vi "TRAMAGGA.vi"(0 "TRAMA":string) -> (1 "Cluster 2":T2, 2 "Cluster":T3, 3 "Cluster 3":T1, 4 "String":string)   [LabVIEW 2020]
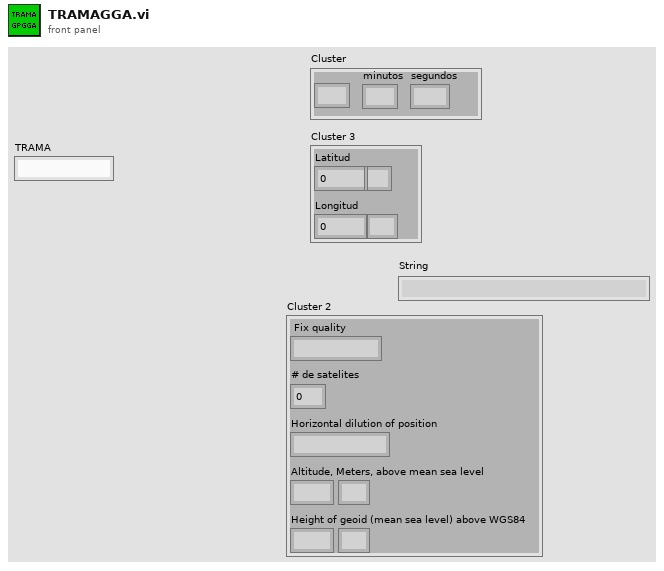
[diagram p1: front panel]
types:
  T1 = cluster{"Latitud":dbl, string, "Longitud":dbl, string}
  T2 = cluster{" Fix quality":string, "# de satelites":dbl, "Horizontal dilution of position":string, "Altitude, Meters, above mean sea level":string, string, "Height of geoid (mean sea level) above WGS84":string, string}
  T3 = cluster{"horas":string, "minutos":string, "segundos ":string}
  T4 = cluster{string, dbl, string, string, string, string, string}
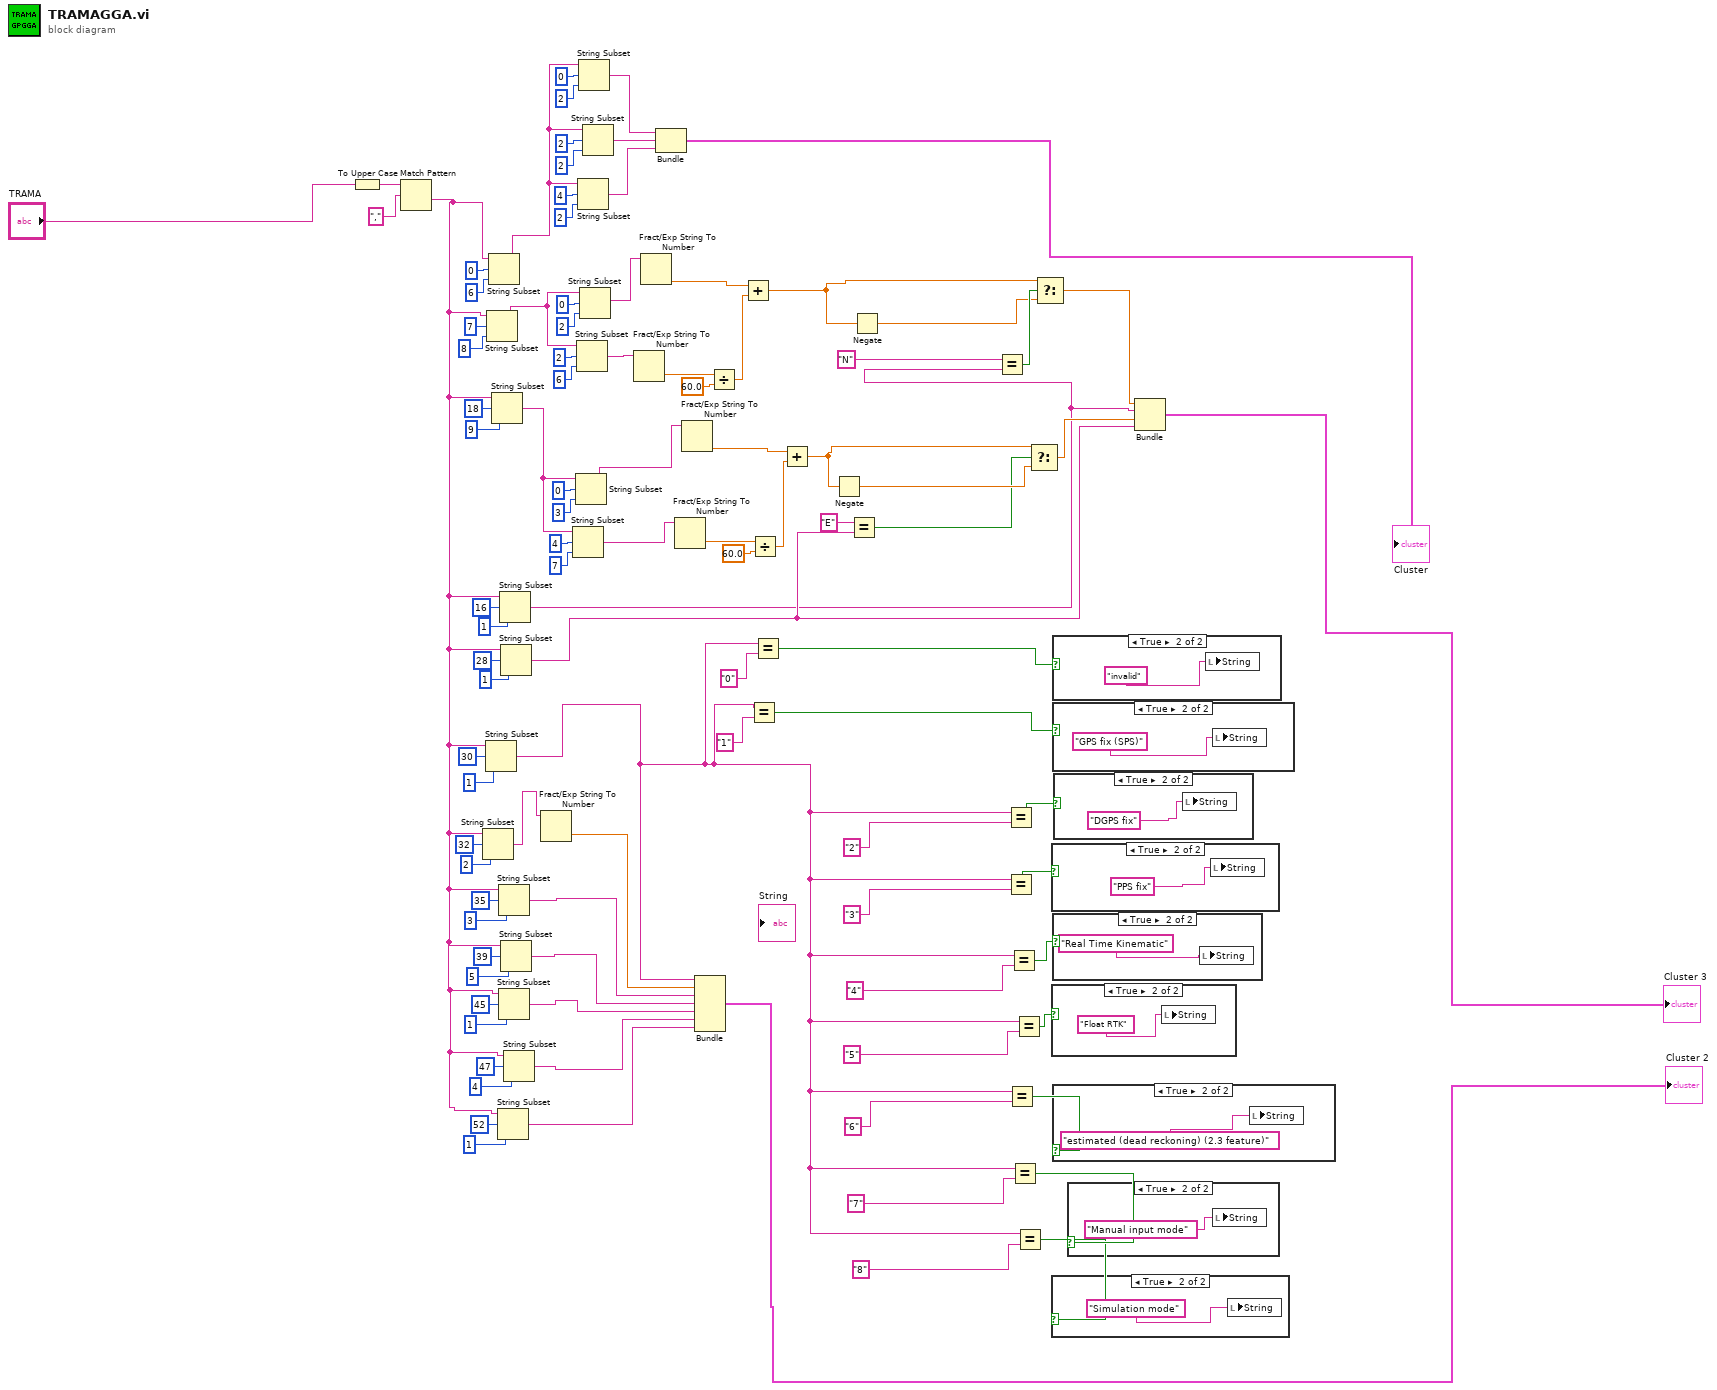
[diagram p0: block diagram]
diagram:
  n1 = To Upper Case(1:"TRAMA") -> (0:w28:string)
  n2 = Match Pattern(string=w28, regular expression=",") -> (after substring=w88:string)  [unwired: 1 in, 3 out]
  n3 = String Subset(string=w88, offset (0)=32, length (rest)=2 ("length (rest)")) -> (substring=w97:string)
  n4 = String Subset(string=w88, offset (0)=30, length (rest)=1 ("length (rest)")) -> (substring=w100:string)
  n5 = String Subset(string=w88, offset (0)=7, length (rest)=8 ("length (rest)")) -> (substring=w25:string)
  n6 = String Subset(string=w88, offset (0)=0, length (rest)=6 ("length (rest)")) -> (substring=w27:string)
  n7 = String Subset(string=w88, offset (0)=18, length (rest)=9 ("length (rest)")) -> (substring=w41:string)
  n8 = String Subset(string=w88, offset (0)=52, length (rest)=1 ("length (rest)")) -> (substring=w94:string)
  n9 = String Subset(string=w88, offset (0)=35, length (rest)=3 ("length (rest)")) -> (substring=w90:string)
  n10 = String Subset(string=w88, offset (0)=45, length (rest)=1 ("length (rest)")) -> (substring=w92:string)
  n11 = String Subset(string=w88, offset (0)=16, length (rest)=1 ("length (rest)")) -> (substring=w49:string)
  n12 = String Subset(string=w88, offset (0)=28, length (rest)=1 ("length (rest)")) -> (substring=w56:string)
  n13 = String Subset(string=w88, offset (0)=39, length (rest)=5 ("length (rest)")) -> (substring=w91:string)
  n14 = String Subset(string=w88, offset (0)=47, length (rest)=4 ("length (rest)")) -> (substring=w93:string)
  n15 = Fract/Exp String To Number(string=w97) -> (number=w89:dbl)  [unwired: 3 in, 1 out]
  n16 = String Subset(string=w41, offset (0)=4, length (rest)=7 ("length (rest)")) -> (substring=w33:string)
  n17 = String Subset(string=w41, offset (0)=0, length (rest)=3 ("length (rest)")) -> (substring=w38:string)
  n18 = String Subset(string=w25, offset (0)=2, length (rest)=6 ("length (rest)")) -> (substring=w12:string)
  n19 = String Subset(string=w27, offset (0)=4, length (rest)=2 ("length (rest)")) -> (substring=w24:string)
  n20 = String Subset(string=w27, offset (0)=0, length (rest)=2 ("length (rest)")) -> (substring=w22:string)
  n21 = String Subset(string=w25, offset (0)=0, length (rest)=2 ("length (rest)")) -> (substring=w15:string)
  n22 = String Subset(string=w27, offset (0)=2, length (rest)=2 ("length (rest)")) -> (substring=w23:string)
  n23 = Fract/Exp String To Number(string=w12) -> (number=w13:dbl)  [unwired: 3 in, 1 out]
  n24 = Fract/Exp String To Number(string=w15) -> (number=w17:dbl)  [unwired: 3 in, 1 out]
  n25 = Bundle(w22, w23, w24) -> (→"Cluster":cluster{string, string, string})  [unwired: 1 in]
  n26 = Fract/Exp String To Number(string=w33) -> (number=w34:dbl)  [unwired: 3 in, 1 out]
  n27 = Fract/Exp String To Number(string=w38) -> (number=w37:dbl)  [unwired: 3 in, 1 out]
  n28 = Bundle(w100, w89, w90, w91, w92, w93, w94) -> (→"Cluster 2":T4)  [unwired: 1 in]
  n29 = Divide(x=w13, y=60.0) -> (x/y=w16:dbl)
  n30 = Add(x=w17, y=w16) -> (x+y=w47:dbl)
  n31 = Equal?(x=w100, y="1") -> (x = y?=w63:bool)
  n32 = Divide(x=w34, y=60.0) -> (x/y=w36:dbl)
  n33 = Equal?(x=w100, y="0") -> (x = y?=w67:bool)
  n34 = Add(x=w37, y=w36) -> (x+y=w55:dbl)
  n35 = Negate(x=w55) -> (-x=w54:dbl)
  n36 = Equal?(x="E", y=w56) -> (x = y?=w52:bool)
  n37 = Negate(x=w47) -> (-x=w48:dbl)
  n38 = Equal?(x="N", y=w49) -> (x = y?=w51:bool)
  n39 = Equal?(x=w100, y="2") -> (x = y?=w69:bool)
  n40 = Equal?(x=w100, y="3") -> (x = y?=w70:bool)
  n41 = Equal?(x=w100, y="6") -> (x = y?=w99:bool)
  n42 = Equal?(x=w100, y="4") -> (x = y?=w72:bool)
  n43 = Equal?(x=w100, y="7") -> (x = y?=w98:bool)
  n44 = Equal?(x=w100, y="5") -> (x = y?=w73:bool)
  n45 = Equal?(x=w100, y="8") -> (x = y?=w74:bool)
  n46 = Select(t=w55, s=w52, f=w54) -> (s? t:f=w57:dbl)
  n47 = Select(t=w47, s=w51, f=w48) -> (s? t:f=w46:dbl)
  n48 = case shown="True" w70 {
    frame False {
    }
    frame True {
      n49 = local write "String"("PPS fix" ("Fix quiality 2")) -> ()
    }
  }
  n50 = case shown="True" w73 {
    frame False {
    }
    frame True {
      n51 = local write "String"("Float RTK" ("Fix quiality 2")) -> ()
    }
  }
  n52 = case shown="True" w74 {
    frame False {
    }
    frame True {
      n53 = local write "String"("Simulation mode" ("Fix quiality 2")) -> ()
    }
  }
  n54 = case shown="True" w67 {
    frame False {
    }
    frame True {
      n55 = local write "String"("invalid" ("Fix quiality 2")) -> ()
    }
  }
  n56 = case shown="True" w63 {
    frame False {
    }
    frame True {
      n57 = local write "String"("GPS fix (SPS)" ("Fix quiality 2")) -> ()
    }
  }
  n58 = case shown="True" w72 {
    frame False {
    }
    frame True {
      n59 = local write "String"("Real Time Kinematic" ("Fix quiality 2")) -> ()
    }
  }
  n60 = case shown="True" w99 {
    frame False {
    }
    frame True {
      n61 = local write "String"("estimated (dead reckoning) (2.3 feature)" ("Fix quiality 2")) -> ()
    }
  }
  n62 = case shown="True" w69 {
    frame False {
    }
    frame True {
      n63 = local write "String"("DGPS fix" ("Fix quiality 2")) -> ()
    }
  }
  n64 = case shown="True" w98 {
    frame False {
    }
    frame True {
      n65 = local write "String"("Manual input mode" ("Fix quiality 2")) -> ()
    }
  }
  n66 = Bundle(w46, w49, w57, w56) -> (→"Cluster 3":cluster{dbl, string, dbl, string})  [unwired: 1 in]
